vi "CAN_CYCLE.vi"(11 "CAN_DATA":T1) -> ()   [LabVIEW 2020, in "ZLG_CAN.lvlib"]
uses:
  ZLG_CAN.lvlib
  Sources/Global_Variable/Global.vi
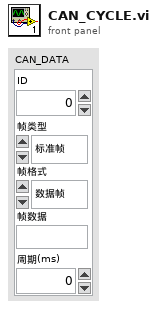
[diagram p1: front panel]
types:
  T1 = cluster{"ID":u32, "帧类型":enum8{"标准帧", "扩展帧"}, "帧格式":enum16{"数据帧", "远程帧"}, "帧数据":string, "周期(ms)":u32}
  T2 = typedef "ZLG_CAN.lvlib/CAN_Frame.ctl" = cluster{"[0]":u8, "[1]":u8, "[2]":u8, "[3]":u8, "[4]":u8, "[5]":u8, "[6]":u8, "[7]":u8}
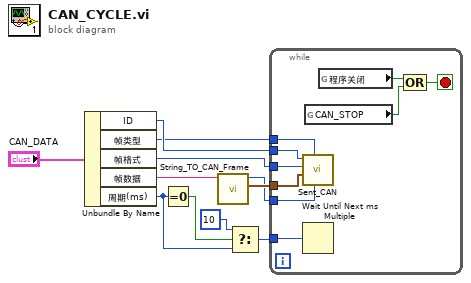
[diagram p0: block diagram]
diagram:
  n1 = Unbundle By Name("CAN_DATA") -> ("ID"=w10:u32, "帧类型"=w9:enum8{"标准帧", "扩展帧"}, "帧格式"=w8:enum16{"数据帧", "远程帧"}, "帧数据"=w7:string, "周期(ms)"=w3:u32)
  n2 = Equal To 0?(x=w3) -> (x = 0?=w4:bool)
  n3 = call "String_TO_CAN_Frame.vi"("CAN_Frame"=w7) -> ("CAN_FRAME"=w6:T2, "DATA_LEN"=w5:i32)  [unwired: 9 in]
  n4 = Select(t=u32 10, s=w4, f=w3) -> (s? t:f=w1:u32)
  n5 = while {
    tunnel: w1 -> [w20]
    tunnel: w10 -> [w19]
    tunnel: w9 -> [w18]
    tunnel: w8 -> [w17]
    tunnel: w6 -> [w15]
    tunnel: w5 -> [w14]
    stop <- w13 stop-if-true
    n6 = call "Sent_CAN.vi"("帧长度"=w14, "帧类型"=w18, "帧数据"=w15, "帧格式"=w17, "ID"=w19) -> ()  [unwired: 6 in, 1 out]
    n7 = Wait Until Next ms Multiple(millisecond multiple=w20) -> ()  [unwired: 1 out]
    n8 = global read "Global.vi" "CAN_STOP"() -> (w12:bool)
    n9 = global read "Global.vi" "程序关闭"() -> (w16:bool)
    n10 = Compound Arithmetic op=OR ("复合运算")(w16, w12) -> (w13:bool)
  }
